vi "poly_robust_unset_cursor_busy_state.vi"(8 "error in (no error)":errorcluster, 9 "disable click? (T)":bool=TRUE) -> (0 "error out":errorcluster, 1 "front pannel is closed?":bool)   [LabVIEW 2015]
uses:
  <vilib>/Utility/error.llb/Clear Errors.vi
  ref_tools/this_vis_name.vi
  ref_tools/polys/poly_this_vis_ref.vi
  ref_tools/name_of_caller.vi
  <vilib>/Utility/cursorutil.llb/Unset Busy.vi
  <vilib>/Utility/cursorutil.llb/Set Busy.vi
  <userlib>/_OpenG.lib/appcontrol/appcontrol.llb/Current VIs Parents Ref__ogtk.vi
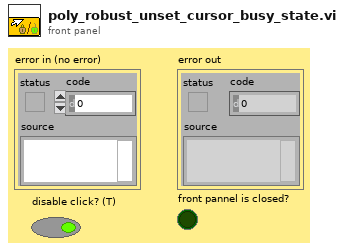
[diagram p1: front panel]
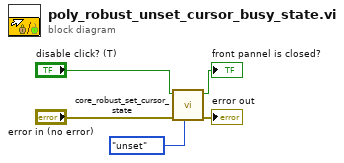
[diagram p0: block diagram]
diagram:
  n1 = call "core_robust_set_cursor_state.vi"("set/unset (set)"=enum16{"set", "unset"}."unset", "error in (no error)"="error in (no error)", "disable click? (T)"="disable click? (T)") -> ("error out"=→"error out":errorcluster, "front pannel is closed?"=→"front pannel is closed?":bool)  [unwired: 7 in]
